vi "Execute Command (Result).vi"(8 "error in (no error)":errorcluster, 9 "Parameter(s)":variant, 10 "SQL":string, 11 "PQ Connection in":refnum<class "PQ Connection.lvclass">) -> (0 "error out":errorcluster, 1 "First Result with Rows returned":refnum<class "PQ Result.lvclass">, 2 "Number of Rows":i32, 3 "PQ Connection out":refnum<class "PQ Connection.lvclass">)   [LabVIEW 2013, in "PQ Connection.lvclass"]
doc: "Execute one or more SQL commands. Optionally, one can provide parameters to be bound to $n tokens in the SQL command (eg. \"SELECT * FROM mytable WHERE x = $1\"). If parameters are provided than only one SQL command can be executed. The parameters can be a cluster or an array, or can be a single value if only one parameter is needed.\n\nThis VI returns a PQ Result object (of the first command to return results, any other reeults are ignored), that can be converted into LabVIEW data. It must be Cleared when it is no longer needed."
uses:
  PQ Connection.lvclass
  Result/PQ Result.lvclass
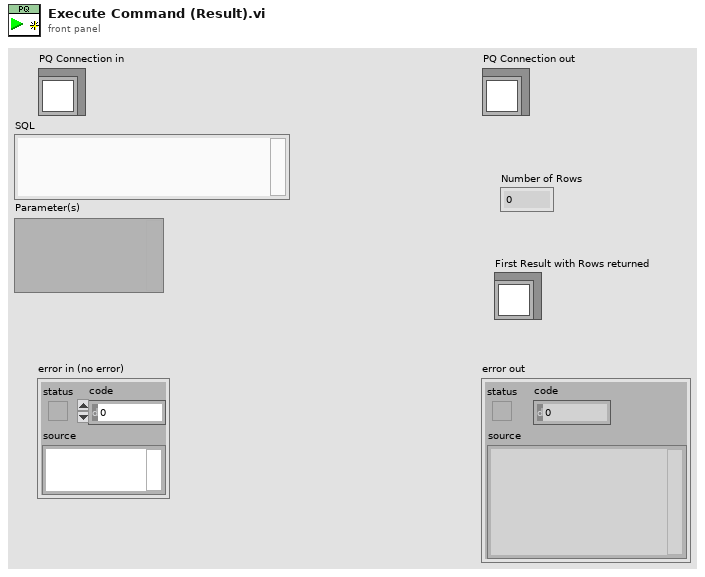
[diagram p1: front panel]
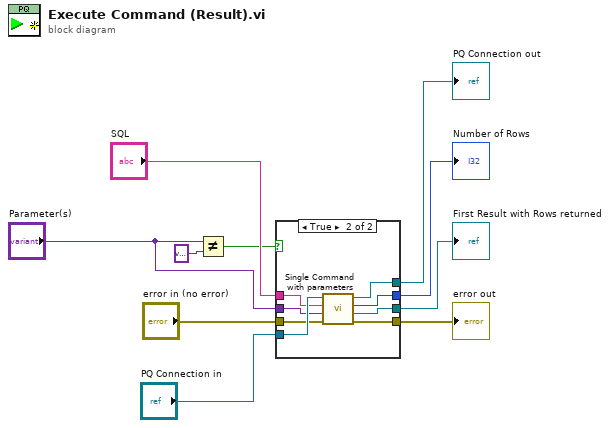
[diagram p0: block diagram]
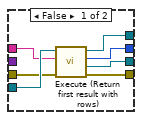
[diagram p2: hidden frame]
diagram:
  n1 = Not Equal?(x="Parameter(s)", y=variant) -> (x != y?=w1:bool)
  n2 = case shown="True" w1 {
    tunnel: "PQ Connection in" -> [w17 w25]
    tunnel: [w16 w24] -> w8
    tunnel: [w15 w23] -> w7
    tunnel: [w14 w22] -> w6
    tunnel: "SQL" -> [w13 w21]
    tunnel: "error in (no error)" -> [w12 w19]
    tunnel: [w11 w18] -> w3
    tunnel: "Parameter(s)" -> [_ w20]
    frame False {
      n3 = call "Execute (Return first result with rows).vi"("error in (no error)"=w12, "SQL"=w13, "PQ Connection in"=w17) -> ("error out"=w11:errorcluster, "First Result with Rows returned"=w15:refnum<class "PQ Result.lvclass">, "Number of Rows"=w14:i32, "PQ Connection out"=w16:refnum<class "PQ Connection.lvclass">)  [unwired: 5 in]
    }
    frame True {
      n4 = call "Single Command with parameters.vi"("error in (no error)"=w19, "Variant (simple type, or Cluster/Array)"=w20, "SQL (Single Command)"=w21, "PQ Connection in"=w25) -> ("error out"=w18:errorcluster, "First Result with Rows returned"=w23:refnum<class "PQ Result.lvclass">, "Number of Rows"=w22:i32, "PQ Connection out"=w24:refnum<class "PQ Connection.lvclass">)  [unwired: 4 in]
    }
  }
  "error out" <- w3
  "PQ Connection out" <- w8
  "First Result with Rows returned" <- w7
  "Number of Rows" <- w6
